vi "Get Channel Values by Block Data Ref.vi"(8 "error in":errorcluster, 9 "Values in":dbl[](array[numeric]), 10 "Block Data Ref in":T1(array[cluster]) {"Data Reference" format="%.0x"}, 11 "Custom Device API in":refnum<class "Custom Device API.lvclass">) -> (0 "error out":errorcluster, 1 "Values out":dbl[](array[numeric]), 2 "Block Data Ref out":T1(array[cluster]) {"Data Reference" format="%.0x"}, 3 "Custom Device API out":refnum<class "Custom Device API.lvclass">)   [LabVIEW 2027, in "Custom Device Interfaces.lvlib" / "Custom Device API.lvclass"]
uses:
  Custom Device API.lvclass
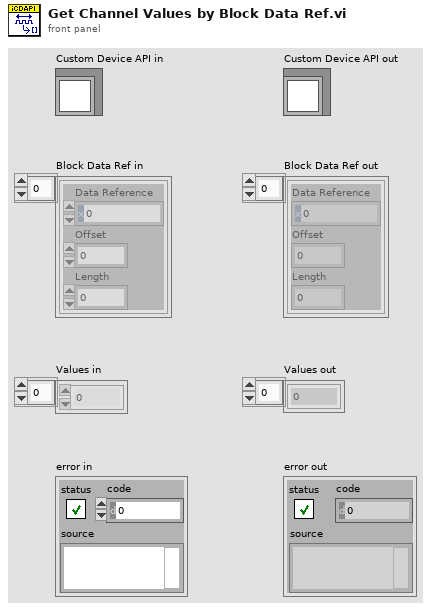
[diagram p1: front panel]
types:
  T1 = cluster{"Data Reference":i32, "Offset":u64, "Length":u64}[]
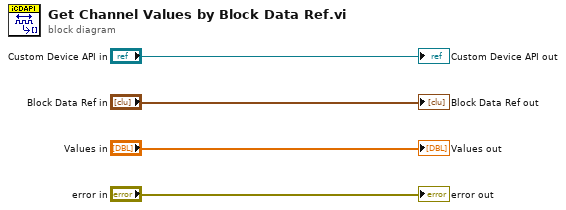
[diagram p0: block diagram]
diagram:
  "error out" <- "error in"
  "Custom Device API out" <- "Custom Device API in"
  "Values out" <- "Values in"
  "Block Data Ref out" <- "Block Data Ref in"
